vi "deploy.vi"(8 "error in (no error)":errorcluster, 10 "build_spec":T1, 11 "lv-builder-l3 in":refnum<class "lv-builder-l3.lvclass">) -> (0 "error out":errorcluster, 3 "lv-builder-l3 out":refnum<class "lv-builder-l3.lvclass">)   [LabVIEW 2015, in "lv-builder-l3.lvlib" / "lv-builder-l3.lvclass"]
uses:
  lv-builder-l3.lvclass
  lv-build/public/_controls/build_specification.ctl
  lv-build/public/_controls/build_type.ctl
  lv-build/lv-build.lvlib
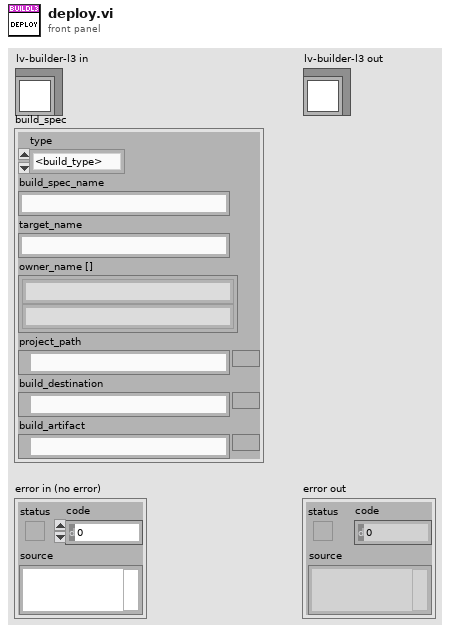
[diagram p1: front panel]
types:
  T1 = typedef "lv-build.lvlib/build_specification.ctl" = cluster{"type":T2, "build_spec_name":string, "target_name":string, "owner_name []":string[], "project_path":path, "build_destination":path, "build_artifact":path}
  T2 = typedef "lv-build.lvlib/build_type.ctl" = enum16{"<build_type>", "application_pc", "application_rt", "installer", "llb", "lvlibp", "zip", "fpga", "<null>"}
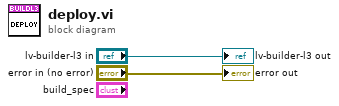
[diagram p0: block diagram]
diagram:
  "error out" <- "error in (no error)"
  "lv-builder-l3 out" <- "lv-builder-l3 in"
